vi "FPGA us.vi"() -> ()   [LabVIEW 2019]
doc: "The myRIO v1.1 FPGA Shipping Personality. This personality contains support for:\n- 2 Analog Input Interrupt channel\n- 4 Digital Input Interrupt channel\n- 1 Timer\n- 1 Accelerometer\n- 1 Button\n- 4 LED\n- 10 Analog Input channels with 1 Sample\n- 6 Analog Output channels with 1 Sample\n- 40 Digital I/O channels with 1 Sample\n- 2 I2C channels\n- 4 Encoder channels\n- 6 PWM channels\n- 2 SPI channels"
uses:
  <vilib>/rvi/Emulation/niFpgaGetClockAttributes.vi
  <vilib>/rvi/Emulation/niFpgaSctlEmulationGetInTimedLoop.vi
  <vilib>/rvi/Emulation/niFpgaEmulationReportErrorSimple.vi
  <vilib>/rvi/eio/common/nirviEmuTemplateMethod_errors.vi
  <vilib>/rvi/Emulation/niFpgaCriticalErrorInLSC.vi
  <vilib>/eio/EIONode/EIONode.xnode
panel:
  out "Meter 3":i16(knob) scale=0.0..10.0
  out "Meter 2":i16(knob) scale=0.0..10.0
  out "Meter":i16(knob) scale=0.0..10.0
  out "Time3":u16
  out "US_L":sgl
  out "US_R":sgl
  out "US_M":sgl
  out "Time1":u16
  out "Time2":u16
  in  "Timeout US":u16
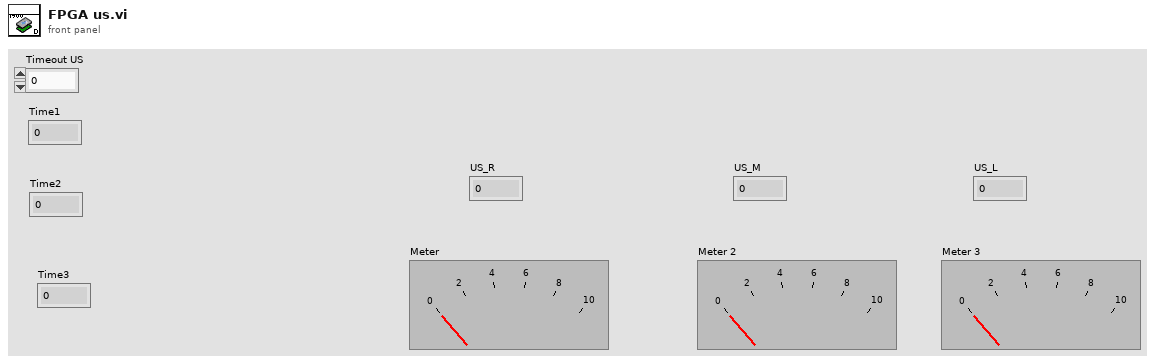
[diagram p1: front panel]
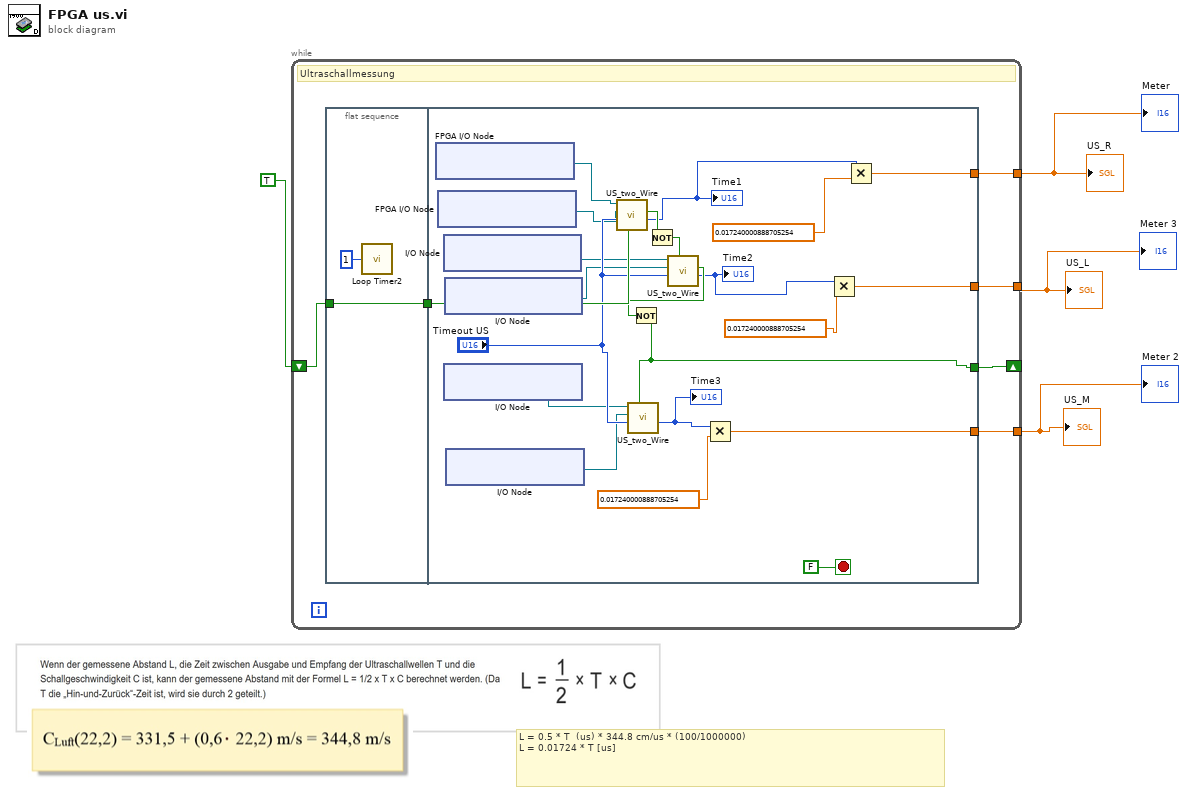
[diagram p0: block diagram]
diagram:
  # "L = 0.5 * T  (us) * 344.8 cm/us * (100/1000000)\nL = 0.01724 * T [us]"
  n1 = while {
    shift-right: [w8] -> _
    shift-left: TRUE -> [w10]
    tunnel: [w7] -> w1
    tunnel: [w6] -> w3
    tunnel: [w5] -> w2
    stop <- FALSE stop-if-true
    # "Ultraschallmessung"
    n2 = flat-sequence {
      tunnel: w10 -> [w12]
      tunnel: [w12] -> w9
      tunnel: w9 -> [w34]
      tunnel: [w14] -> w8
      tunnel: [w22] -> w7
      tunnel: [w19] -> w6
      tunnel: [w16] -> w5
      frame #0 {
        n3 = call "Loop Timer2"("Count(uSec)"=u16 1 ("Count(Ticks)")) -> ()  [unwired: 1 out]
      }
      frame #1 {
        n4 = xnode "FPGA I/O Node"() -> ("FPGA I/O Out"=w29:refnum<k21>)  [unwired: 1 in, 1 out]
        n5 = xnode "FPGA I/O Node"() -> ("FPGA I/O Out"=w28:refnum<k21>)  [unwired: 1 in, 1 out]
        n6 = xnode ("I/O Node")() -> ("FPGA I/O Out"=w27:refnum<k21>)  [unwired: 1 in, 1 out]
        n7 = xnode ("I/O Node")() -> ("FPGA I/O Out"=w25:refnum<k21>)  [unwired: 1 in, 1 out]
        n8 = xnode ("I/O Node")() -> ("FPGA I/O Out"=w26:refnum<k21>)  [unwired: 1 in, 1 out]
        n9 = xnode ("I/O Node")() -> ("FPGA I/O Out"=w24:refnum<k21>)  [unwired: 1 in, 1 out]
        n10 = call "US_two_Wire.vi"("start ping"=w34, "Timeout (usec)"="Timeout US", "Echo_Line"=w28, "Ping_Line"=w29) -> ("echo_time(us)"=w21:u16, "busy"=w32:bool)  [unwired: 6 in]
        "Time1" <- w21
        n11 = Not(x=w32) -> (.not. x?=w33:bool)
        n12 = call "US_two_Wire.vi"("start ping"=w33, "Timeout (usec)"="Timeout US", "Echo_Line"=w26, "Ping_Line"=w27) -> ("echo_time(us)"=w18:u16, "busy"=w31:bool)  [unwired: 6 in]
        "Time2" <- w18
        n13 = Not(x=w31) -> (.not. x?=w14:bool)
        n14 = call "US_two_Wire.vi"("start ping"=w14, "Timeout (usec)"="Timeout US", "Echo_Line"=w24, "Ping_Line"=w25) -> ("echo_time(us)"=w15:u16)  [unwired: 6 in, 1 out]
        "Time3" <- w15
        n15 = Multiply(x=w15, y=sgl 0.01724) -> (x*y=w22:sgl)
        n16 = Multiply(x=w18, y=sgl 0.01724) -> (x*y=w16:sgl)
        n17 = Multiply(x=w21, y=sgl 0.01724) -> (x*y=w19:sgl)
      }
    }
  }
  "US_M" <- w1
  "US_R" <- w3
  "US_L" <- w2
  "Meter 3" <- w2
  "Meter 2" <- w1
  "Meter" <- w3
